vi "interface_Init.vi"(0 "object in":refnum<class "interface.lvclass">, 5 "error in (no error)":errorcluster) -> (14 "object out":refnum<class "interface.lvclass">, 15 "configout":T1, 19 "error out":errorcluster)   [LabVIEW 2016, in "interface.lvclass"]
uses:
  interface.lvclass
  <vilib>/Utility/config.llb/NI_LVConfig.lvlib
panel:
  in  "参数数值":T2={"CODMn"=TRUE, "CODCr"=TRUE, "DO"=TRUE, "铜"=TRUE, "PH"=TRUE, "氨氮"=TRUE, "比电导率"=TRUE, "水温"=TRUE, "COD"=TRUE, "浊度"=TRUE, "总氮"=TRUE, "总磷"=TRUE, "叶绿素a"=TRUE, "藻密度"=TRUE, "水位"=TRUE, "流速"=TRUE, "瞬时流量"=TRUE, "累积流量"=TRUE, "亚硝氮"=TRUE, "硫化物"=TRUE, "ORP"=TRUE, "铅"=TRUE, "镉"=TRUE, "锌"=TRUE, "镍"=TRUE, "锰"=TRUE, "汞"=TRUE, "气温"=TRUE, "气压"=TRUE, "风速"=TRUE, "风向"=TRUE, "盐度"=TRUE, "磷酸盐"=TRUE, "硝氮"=TRUE, "氟化物"=TRUE, "挥发酚"=TRUE, "氯化物"=TRUE}
  out "配置表格":string[][](table)
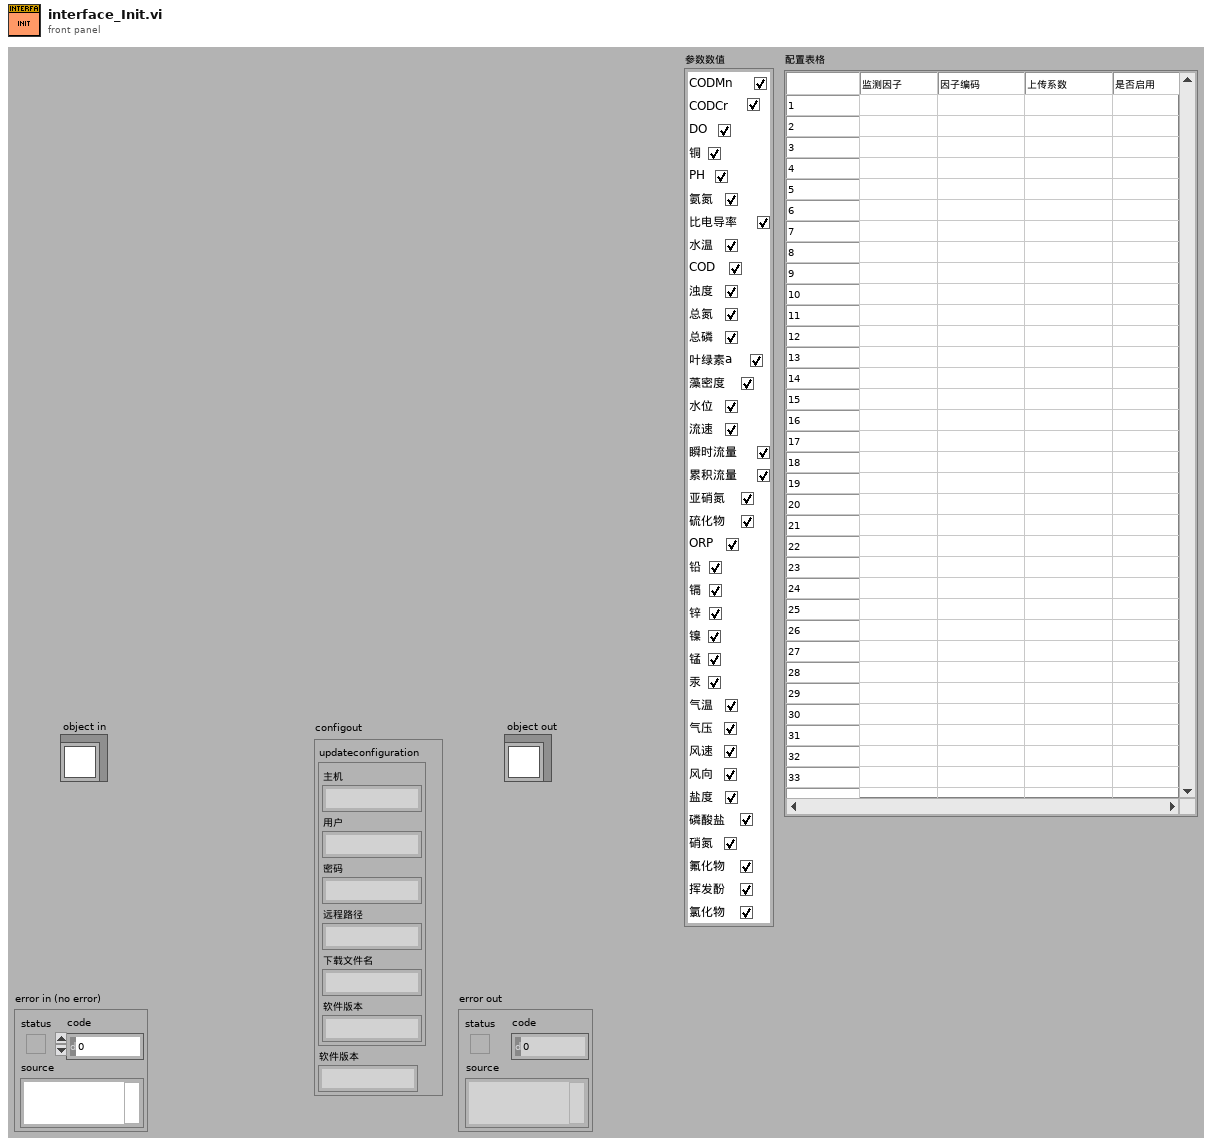
[diagram p1: front panel]
types:
  T1 = cluster{"updateconfiguration":cluster{"主机":string, "用户":string, "密码":string, "远程路径":string, "下载文件名":string, "软件版本":string}, "软件版本":string}
  T2 = cluster{"CODMn":bool, "CODCr":bool, "DO":bool, "铜":bool, "PH":bool, "氨氮":bool, "比电导率":bool, "水温":bool, "COD":bool, "浊度":bool, "总氮":bool, "总磷":bool, "叶绿素a":bool, "藻密度":bool, "水位":bool, "流速":bool, "瞬时流量":bool, "累积流量":bool, "亚硝氮":bool, "硫化物":bool, "ORP":bool, "铅":bool, "镉":bool, "锌":bool, "镍":bool, "锰":bool, "汞":bool, "气温":bool, "气压":bool, "风速":bool, "风向":bool, "盐度":bool, "磷酸盐":bool, "硝氮":bool, "氟化物":bool, "挥发酚":bool, "氯化物":bool}
  T3 = typedef "NI_LVConfig.lvlib/Config Data RefNum.ctl" = refnum<k1>
  T4 = cluster{"主机":string, "用户":string, "密码":string, "远程路径":string, "下载文件名":string, "软件版本":string}
  T5 = cluster{"updateconfiguration":cluster{"主机":string, "用户":string, "密码":string, "远程路径":string, "下载文件名":string, "软件版本":string}, string}
  T6 = cluster{"[0]":string, "[1]":string, "[2]":string, "[3]":string, "[4]":string, "[5]":string, "[6]":string, "[7]":string, "[8]":string, "[9]":string, "[10]":string, "[11]":string, "[12]":string, "[13]":string, "[14]":string, "[15]":string, "[16]":string, "[17]":string, "[18]":string, "[19]":string, "[20]":string, "[21]":string, "[22]":string, "[23]":string, "[24]":string, "[25]":string, "[26]":string, "[27]":string, "[28]":string, "[29]":string, "[30]":string, "[31]":string, "[32]":string, "[33]":string, "[34]":string, "[35]":string, "[36]":string}
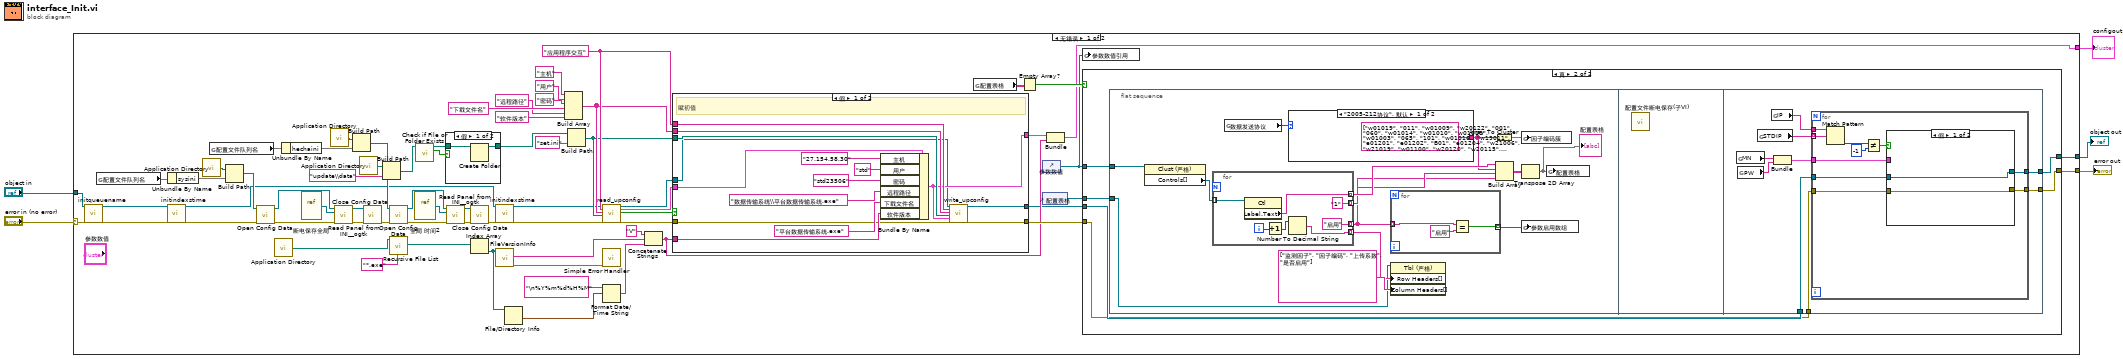
[diagram p0: block diagram]
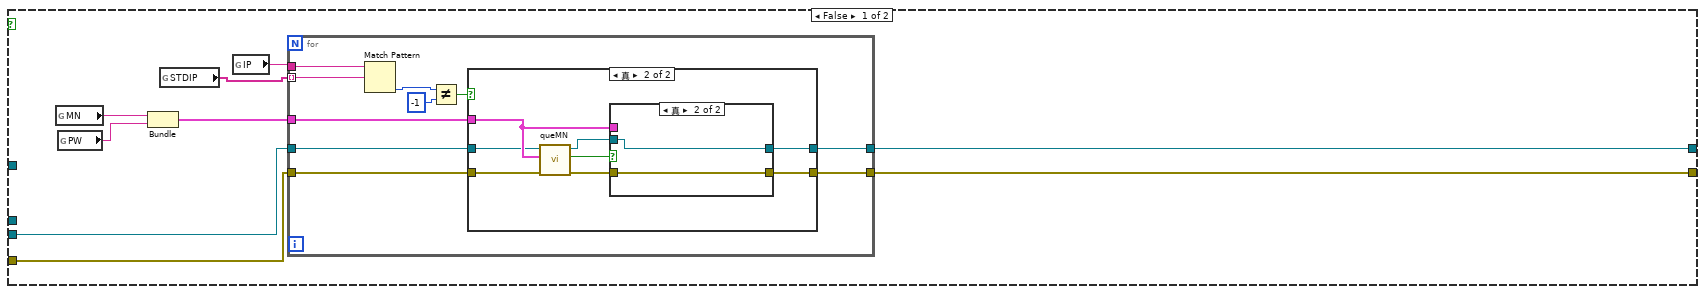
[diagram p2: hidden frame]
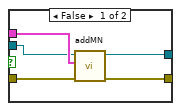
[diagram p4: hidden frame]
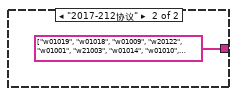
[diagram p5: hidden frame]
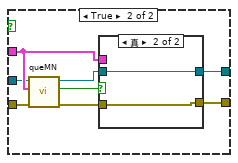
[diagram p6: hidden frame]
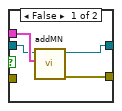
[diagram p7: hidden frame]
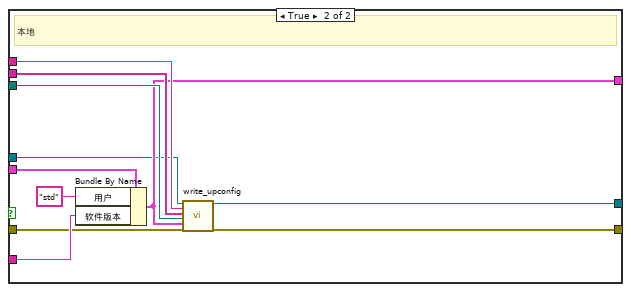
[diagram p9: hidden frame]
diagram:
  n1 = case shown="无错误" "error in (no error)" {
    selector: "error in (no error)" -> [w72 w207]
    tunnel: "object in" -> [w74 w208]
    tunnel: [w11 w208] -> w3
    tunnel: [w13 w207] -> w2
    tunnel: [w6 _] -> w1
    frame No Error {
      w29 = "应用程序交互" ("section")
      n2 = call-dynamic "initqueuename.vi"("object in"=w74, "error in (no error)"=w72) -> ("object out"=w73:refnum<class "interface.lvclass">, "error out"=w71:errorcluster)  [unwired: 16 in]
      n3 = global read "断电保存全局.vi" "配置文件队列名"() -> (w67)
      n4 = Unbundle By Name(w67) -> ("sysini"=w68)
      n5 = call-dynamic "initindexstime.vi"("object in"=w73, "error in (no error)"=w71) -> ("object out"=w10:refnum<class "interface.lvclass">, "error out"=w14:errorcluster)  [unwired: 16 in]
      n6 = call <vilib>:"Application Directory.vi"() -> ("Application Directory"=w43:path)
      n7 = global read "断电保存全局.vi" "配置文件队列名"() -> (w69)
      n8 = Build Path(base path=w43, name or relative path=w68) -> (appended path=w44:path)
      n9 = call <vilib>:"Open Config Data.vi"("error in (no error)"=w14, "configuration file path"=w44) -> ("error out"=w39:errorcluster, "refnum"=w40:T3)  [unwired: 7 in, 1 out]
      n10 = call <vilib>:"Application Directory.vi"() -> ("Application Directory"=w37:path)
      n11 = Unbundle By Name(w69) -> ("hechaini"=w70)
      n12 = vi-ref "断电保存全局.vi"() -> (w41:refnum<vi>)
      n13 = call <vilib>:"Application Directory.vi"() -> ("Application Directory"=w49:path)
      n14 = call <userlib>:"Read Panel from INI__ogtk.vi"("error in (no error)"=w39, "VI ref"=w41, "refnum"=w40) -> ("error out"=w45:errorcluster, "refnum out"=w42:T3)  [unwired: 7 in]
      n15 = Build Path(base path=w49, name or relative path=w70) -> (appended path=w48:path)
      n16 = call <vilib>:"Application Directory.vi"() -> ("Application Directory"=w64:path)
      n17 = call <vilib>:"Close Config Data.vi"("error in (no error)"=w45, "refnum"=w42) -> ("error out"=w19:errorcluster)  [unwired: 8 in, 1 out]
      n18 = Build Path(base path=w64, name or relative path="update\\data" ("名称或相对路径")) -> (appended path=w63:path)
      n19 = call <vilib>:"Open Config Data.vi"("error in (no error)"=w19, "configuration file path"=w48) -> ("error out"=w53:errorcluster, "refnum"=w52:T3)  [unwired: 7 in, 1 out]
      n20 = call <vilib>:"Recursive File List.vi"("pattern"="*.exe", "Folder Path"=w37) -> ("All Files in Dir"=w31:path[])  [unwired: 5 in, 4 out]
      n21 = vi-ref "全局 时间2.vi"() -> (w51:refnum<vi>)
      n22 = call <vilib>:"Check if File or Folder Exists.vi"("path"=w63) -> ("file or folder exists?"=w62:bool, "dup path"=w61:path)  [unwired: 8 in, 1 out]
      n23 = case shown="假" w62 {
        tunnel: w61 -> [w179 w180]
        tunnel: [w178 w180] -> w66
        frame False {
          n24 = Create Folder(path (use dialog)=w179) -> (created path=w178:path)  [unwired: 2 in, 2 out]
        }
        frame True {
        }
      }
      n25 = call <userlib>:"Read Panel from INI__ogtk.vi"("error in (no error)"=w53, "VI ref"=w51, "refnum"=w52) -> ("error out"=w54:errorcluster, "refnum out"=w50:T3)  [unwired: 7 in]
      n26 = call <vilib>:"Close Config Data.vi"("error in (no error)"=w54, "refnum"=w50) -> ("error out"=w22:errorcluster)  [unwired: 8 in, 1 out]
      n27 = Index Array(array=w31) -> (element=w32:path)  [unwired: 1 in]
      n28 = call-dynamic "initindexstime.vi"("object in"=w10, "error in (no error)"=w22) -> ("object out"=w21:refnum<class "interface.lvclass">, "error out"=w20:errorcluster)  [unwired: 16 in]
      n29 = call <vilib>:"FileVersionInfo.vi"("Application Path in"=w32) -> ("error out"=w38:errorcluster, "File Version Info"=w47:string)  [unwired: 7 in, 2 out]
      n30 = File/Directory Info(path=w32) -> (last mod=w33:timestamp)  [unwired: 1 in, 6 out]
      n31 = Build Array("主机" ("section"), "用户" ("section"), "密码" ("key"), "远程路径" ("key"), "下载文件名" ("key"), "软件版本" ("key")) -> (w28:string[])
      n32 = Build Path(base path=w66, name or relative path="set.ini" ("名称或相对路径")) -> (appended path=w27:path)
      n33 = call-dynamic "read_upconfig.vi"("object in"=w21, "段"=w29, "键数组"=w28, "configuration file path"=w27, "error in (no error)"=w20) -> ("object out"=w23:refnum<class "interface.lvclass">, "updateconfiguration"=w26:T4, "section exists?"=w25:bool, "error out"=w24:errorcluster)  [unwired: 11 in]
      n34 = call <vilib>:"Simple Error Handler.vi"("error in (no error)"=w38) -> ()  [unwired: 4 in, 5 out]
      n35 = Format Date/Time String(time format string (%c)="\n%Y%m%d%H%M" ("时间格式字符串(%c)"), seconds (now)=w33) -> (date/time string=w36:string)  [unwired: 1 in]
      n36 = Concatenate Strings("V" ("字符串"), w47, w36) -> (w8:string)
      n37 = case shown="假" w25 {
        tunnel: w26 -> [w194 w205]
        tunnel: [w185 w199] -> w9
        tunnel: w8 -> [w189 w206]
        tunnel: w29 -> [w188 w203]
        tunnel: w28 -> [w187 w202]
        tunnel: w27 -> [w186 w201]
        tunnel: w24 -> [w183 w200]
        tunnel: w23 -> [w184 w197]
        tunnel: [w182 w198] -> w7
        tunnel: [w181 w196] -> w12
        frame False {
          # "赋初值"
          n38 = Bundle By Name(cluster=w194, "主机"="27.154.58.30" ("key"), "用户"="std", "密码"="std23506", "远程路径"="数据传输系统\\平台数据传输系统.exe", "下载文件名"="平台数据传输系统.exe", "软件版本"=w189) -> (w185:T4)
          n39 = call-dynamic "write_upconfig.vi"("object in"=w184, "段"=w188, "键数组"=w187, "configuration file path"=w186, "updateconfiguration"=w185, "error in (no error)"=w183) -> ("object out"=w182:refnum<class "interface.lvclass">, "error out"=w181:errorcluster)  [unwired: 12 in]
        }
        frame True {
          # "本地"
          n40 = Bundle By Name(cluster=w205, "用户"="std", "软件版本"=w206) -> (w199:T4)
          n41 = call-dynamic "write_upconfig.vi"("object in"=w197, "段"=w203, "键数组"=w202, "configuration file path"=w201, "updateconfiguration"=w199, "error in (no error)"=w200) -> ("object out"=w198:refnum<class "interface.lvclass">, "error out"=w196:errorcluster)  [unwired: 12 in]
        }
      }
      n42 = global read "断电保存全局.vi" "配置表格"() -> (w17:string[][])
      n43 = Empty Array?(array=w17) -> (empty?=w16:bool)
      n44 = control-ref of="参数数值"() -> (w15:refnum<vi>)
      n45 = control-ref of="配置表格"() -> (w18:refnum<vi>)
      n46 = Bundle("updateconfiguration"=w9, w8) -> (w6:T5)  [unwired: 1 in]
      n47 = global write "断电保存全局.vi" "参数数值引用"(w15) -> ()
      n48 = case shown="真" w16 {
        tunnel: w18 -> [_ w116]
        tunnel: w15 -> [_ w115]
        tunnel: w7 -> [w78 w114]
        tunnel: w12 -> [w77 w113]
        tunnel: [w76 w112] -> w11
        tunnel: [w75 w111] -> w13
        frame False {
          n49 = global read "断电保存全局.vi" "MN"() -> (w83:string)
          n50 = global read "断电保存全局.vi" "PW"() -> (w82:string)
          n51 = Bundle("MN"=w83, "PW"=w82) -> (w81:cluster{"MN":string, "PW":string})  [unwired: 1 in]
          n52 = global read "断电保存全局.vi" "STDIP"() -> (w80:string[])
          n53 = global read "断电保存全局.vi" "IP"() -> (w79:string)
          n54 = for {
            tunnel: w80 -> [w93] mode=indexing
            tunnel: w79 -> [w92]
            tunnel: w81 -> [w88]
            tunnel: w78 -> [w87]
            tunnel: w77 -> [w86]
            tunnel: [w85] -> w76
            tunnel: [w84] -> w75
            n55 = Match Pattern(string=w92, regular expression=w93) -> (offset past match=w91:i32)  [unwired: 1 in, 3 out]
            n56 = Not Equal?(x=w91, y=-1) -> (x != y?=w89:bool)
            n57 = case shown="真" w89 {
              tunnel: w88 -> [_ w103]
              tunnel: w87 -> [w95 w101]
              tunnel: w86 -> [w94 w100]
              tunnel: [w95 w98] -> w85
              tunnel: [w94 w96] -> w84
              frame False {
              }
              frame True {
                n58 = call "queMN.vi"("error in (no error)"=w100, "簇"=w103, "interface 输入"=w101) -> ("error out"=w97:errorcluster, "包含启动项"=w102:bool, "interface 输出"=w99:refnum<class "interface.lvclass">)  [unwired: 6 in]
                n59 = case shown="真" w102 {
                  tunnel: w103 -> [w108 _]
                  tunnel: w99 -> [w107 w110]
                  tunnel: [w106 w110] -> w98
                  tunnel: w97 -> [w105 w109]
                  tunnel: [w104 w109] -> w96
                  frame False {
                    n60 = call "addMN.vi"("error in (no error)"=w105, "簇"=w108, "interface 输入"=w107) -> ("error out"=w104:errorcluster, "interface 输出"=w106:refnum<class "interface.lvclass">)  [unwired: 6 in, 1 out]
                  }
                  frame True {
                  }
                }
              }
            }
          }
        }
        frame True {
          n61 = flat-sequence {
            tunnel: w116 -> [w118]
            tunnel: w115 -> [w117]
            tunnel: w114 -> [w146]
            tunnel: w113 -> [w145]
            tunnel: [w144] -> w112
            tunnel: [w143] -> w111
            frame #0 {
              n62 = property on="属性节点" class="Clust (严格)"(reference=w117) -> ("Controls[]"=w126:refnum<vi>[])  [unwired: 1 in, 2 out]
              n63 = for {
                tunnel: w126 -> [w142] mode=indexing
                tunnel: [w141] -> w128 mode=indexing
                tunnel: [w139] -> w127 mode=indexing
                tunnel: ["1"] -> w121 mode=indexing
                tunnel: ["启用"] -> w120 mode=indexing
                i -> [w140]
                n64 = property class="Ctl"(reference=w142) -> ("Label.Text"=w141:string)  [unwired: 1 in, 2 out]
                n65 = Increment(x=w140) -> (x+1=w138:i32)
                n66 = Number To Decimal String(number=w138) -> (decimal integer string=w139:string)  [unwired: 1 in]
              }
              n67 = global read "断电保存全局.vi" "数据发送协议"() -> (w124:enum16{"2005-212协议", "2017-212协议"})
              n68 = case shown="\"2005-212协议\", 默认" w124 {
                tunnel: [string[] ["w01019", "011", "w01009", "w20122", "001", "060", "w01014", "w01010", "w01018", "w01003", "065", "101", "w01016", "w19011", "e01201", "e01202", "B01", "e01204", "w21006", "w21019", "w01100", "w20120", "w20115", "w20123", "w20121", "w20124", "w20111", "a01001", "a01006", "a01007", "a01008", "w01002", "w21015", "w21007", "w21017", "w23002", "w21002"] string[] ["w01019", "w01018", "w01009", "w20122", "w01001", "w21003", "w01014", "w01010", "w01018", "w01003", "w21001", "w21011", "w01016", "w19011", "e01201", "e01202", "e01203", "e01204", "w21006", "w21019", "w01100", "w20120", "w20115", "w20123", "w20121", "w20124", "w20111", "a01001", "a01006", "a01007", "a01008", "w01002", "w21015", "w21007", "w21017", "w23002", "w21002"]] -> w122
                frame "2005-212协议", Default {
                }
                frame "2017-212协议" {
                }
              }
              n69 = for {
                tunnel: w120 -> [w133] mode=indexing
                tunnel: [w131] -> w119 mode=indexing
                n70 = Equal?(x=w133, y="启用") -> (x = y?=w131:bool)
              }
              n71 = property on="属性节点" class="Tbl (严格)"(reference=w118, "Row Headers[]"=w127, "Column Headers[]"=string[] ["监测因子", "因子编码", "上传系数", "是否启用"]) -> ()  [unwired: 1 in, 2 out]
              n72 = Array To Cluster(array=w122) -> (cluster=w123:T6)
              n73 = Build Array(w128, w122, w121, w120) -> (w130:string[][])
              n74 = global write "断电保存全局.vi" "因子编码簇"(w123) -> ()
              n75 = Transpose 2D Array(2D array=w130) -> (transposed array=w125:string[][])
              "配置表格" <- w125
              n76 = global write "断电保存全局.vi" "参数启用数组"(w119) -> ()
              n77 = global write "断电保存全局.vi" "配置表格"(w125) -> ()
            }
            frame #1 {
              n78 = call "配置文件断电保存(子VI).vi"() -> ()  [unwired: 12 in]
            }
            frame #2 {
              n79 = global read "断电保存全局.vi" "MN"() -> (w151:string)
              n80 = global read "断电保存全局.vi" "PW"() -> (w150:string)
              n81 = global read "断电保存全局.vi" "STDIP"() -> (w148:string[])
              n82 = global read "断电保存全局.vi" "IP"() -> (w147:string)
              n83 = Bundle("MN"=w151, "PW"=w150) -> (w149:cluster{"MN":string, "PW":string})  [unwired: 1 in]
              n84 = for {
                tunnel: w148 -> [w161] mode=indexing
                tunnel: w147 -> [w160]
                tunnel: w149 -> [w157]
                tunnel: w146 -> [w155]
                tunnel: w145 -> [w154]
                tunnel: [w153] -> w144
                tunnel: [w152] -> w143
                n85 = Match Pattern(string=w160, regular expression=w161) -> (offset past match=w159:i32)  [unwired: 1 in, 3 out]
                n86 = Not Equal?(x=w159, y=-1) -> (x != y?=w156:bool)
                n87 = case shown="假" w156 {
                  tunnel: w157 -> [_ w171]
                  tunnel: w155 -> [w163 w169]
                  tunnel: w154 -> [w162 w168]
                  tunnel: [w163 w166] -> w153
                  tunnel: [w162 w165] -> w152
                  frame False {
                  }
                  frame True {
                    n88 = call "queMN.vi"("error in (no error)"=w168, "簇"=w171, "interface 输入"=w169) -> ("error out"=w164:errorcluster, "包含启动项"=w170:bool, "interface 输出"=w167:refnum<class "interface.lvclass">)  [unwired: 6 in]
                    n89 = case shown="真" w170 {
                      tunnel: w171 -> [w175 _]
                      tunnel: w167 -> [w174 w177]
                      tunnel: [w173 w177] -> w166
                      tunnel: [w172 w176] -> w165
                      tunnel: w164 -> [_ w176]
                      frame False {
                        n90 = call "addMN.vi"("簇"=w175, "interface 输入"=w174) -> ("error out"=w172:errorcluster, "interface 输出"=w173:refnum<class "interface.lvclass">)  [unwired: 7 in, 1 out]
                      }
                      frame True {
                      }
                    }
                  }
                }
              }
            }
          }
        }
      }
    }
    frame Error {
    }
  }
  "object out" <- w3
  "error out" <- w2
  "configout" <- w1
